vi "simx Get Ping Time.vi"(8 "error in (no error)":errorcluster, 10 "pingTime":i32, 11 "clientID":i32) -> (0 "error out":errorcluster, 2 "pingTime out":i32, 3 "function return":i32)   [LabVIEW 2019, in "PXL_V-REP.lvlib"]
doc: "EXTAPI_DLLEXPORT simxInt simxGetPingTime(simxInt clientID,simxInt* pingTime);"
uses:
  PXL_V-REP.lvlib
  <userlib>/V-REP/remoteApi.dll
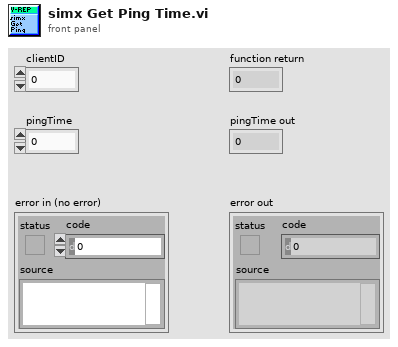
[diagram p1: front panel]
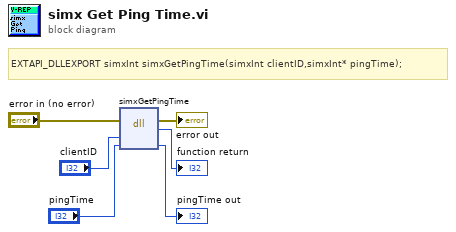
[diagram p0: block diagram]
diagram:
  # "EXTAPI_DLLEXPORT simxInt simxGetPingTime(simxInt clientID,simxInt* pingTime);"
  n1 = dll-call lib="C:/Program Files (x86)/National Instruments/LabVIEW 2019/user.lib/V-REP/remoteApi.*" fn="simxGetPingTime"(error in="error in (no error)", "clientID"="clientID", "pingTime"="pingTime") -> (error out=→"error out":errorcluster, →"function return":i32, "pingTime"=→"pingTime out":i32)  [unwired: 3 in, 1 out]
